vi "Com Read.vi"(8 "错误输入（无错误）":errorcluster, 9 "num":u32, 10 "超时":u32, 11 "VISA In":refnum<visa-resource-name>) -> (0 "错误输出":errorcluster, 1 "END":string, 2 "buff":string, 3 "VISA Out":refnum<visa-resource-name>)   [LabVIEW 2015, in "WZ5005E.lvlib"]
uses:
  WZ5005E.lvlib
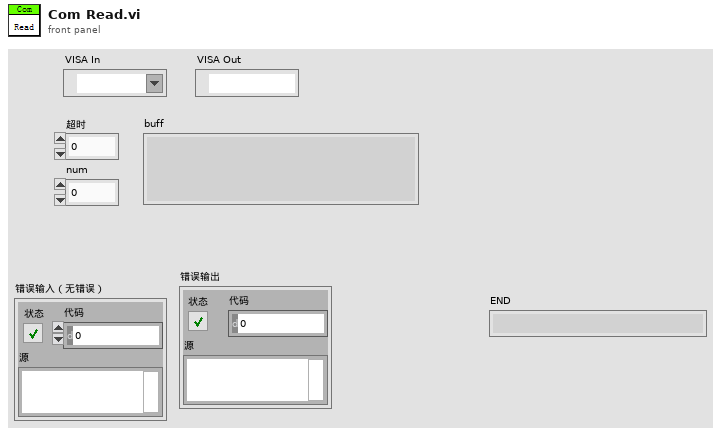
[diagram p1: front panel]
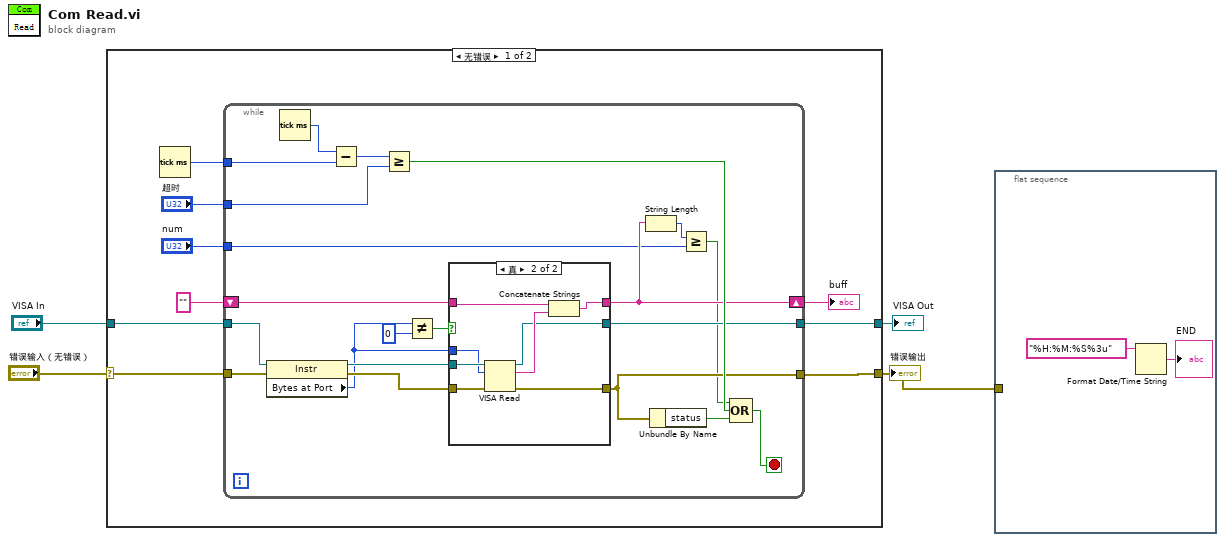
[diagram p0: block diagram]
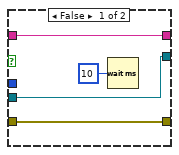
[diagram p2: hidden frame]
diagram:
  n1 = case shown="无错误" "错误输入（无错误）" {
    selector: "错误输入（无错误）" -> [w13 w48]
    tunnel: "VISA In" -> [w12 w47]
    tunnel: [w7 w48] -> w1
    tunnel: [w8 w47] -> w2
    frame No Error {
      n2 = Tick Count (ms)() -> (millisecond timer value=w11:u32)
      n3 = while {
        tunnel: w13 -> [w33]
        tunnel: w12 -> [w34]
        tunnel: w11 -> [w28]
        tunnel: "超时" -> [w26]
        shift-right: [w18] -> w5
        shift-left: "" -> [w22]
        tunnel: [w21] -> w8
        tunnel: [w19] -> w7
        tunnel: "num" -> [w16]
        stop <- w25 stop-if-true
        n4 = property class="Instr"(reference=w34, error in=w33) -> (reference out=w30:refnum<visa-resource-name>, error out=w20:errorcluster, "Bytes at Port"=w14:u32)
        n5 = Tick Count (ms)() -> (millisecond timer value=w29:u32)
        n6 = Subtract(x=w29, y=w28) -> (x-y=w27:u32)
        n7 = Greater Or Equal?(x=w27, y=w26) -> (x >= y?=w24:bool)
        n8 = Not Equal?(x=w14, y=u32 0) -> (x != y?=w31:bool)
        n9 = case shown="真" w31 {
          tunnel: w30 -> [w37 w46]
          tunnel: [w36 w45] -> w19
          tunnel: w22 -> [w35 w44]
          tunnel: [w35 w42] -> w18
          tunnel: [w37 w41] -> w21
          tunnel: w20 -> [w36 w40]
          tunnel: w14 -> [_ w39]
          frame False {
            n10 = Wait (ms)(milliseconds to wait=u32 10 ("等待时间（毫秒）")) -> ()  [unwired: 1 out]
          }
          frame True {
            n11 = VISA Read(VISA resource name=w46, byte count=w39, error in (no error)=w40) -> (VISA resource name out=w41:refnum<visa-resource-name>, read buffer=w43:string, error out=w45:errorcluster)  [unwired: 1 out]
            n12 = Concatenate Strings(w44, w43) -> (w42:string)
          }
        }
        n13 = String Length(string=w18) -> (length=w17:i32)
        n14 = Unbundle By Name(w19) -> ("status"=w23:bool)
        n15 = Greater Or Equal?(x=w17, y=w16) -> (x >= y?=w15:bool)
        n16 = Compound Arithmetic op=OR ("复合运算")(w15, w24, w23) -> (w25:bool)
      }
      "buff" <- w5
    }
    frame Error {
    }
  }
  "错误输出" <- w1
  "VISA Out" <- w2
  n17 = flat-sequence {
    tunnel: w1 -> [_]
    frame #0 {
      n18 = Format Date/Time String(time format string (%c)="%H:%M:%S%3u" ("时间格式字符串(%c)")) -> (date/time string=→"END":string)  [unwired: 2 in]
    }
  }
